vi "PDF HovaCAL fix Tables.vi"(8 "Sprachliste":string[][](array[string])) -> (2 "Bemerkungen":string[](array[string]), 3 "Eingabetabelle behandelt":string[][][](array[string]))   [LabVIEW 2020, in "Linearisierung v2.lvlib" / "Protokoll.lvlib"]
uses:
  Protokoll.lvlib
  Gasteiler/HovaCAL_Interface/Kommunikation/Aktion FGV HovaCAL Interface Autolin.ctl
  Visualisierungs Elemente/String - Ausgabefeld.ctl
  Seiten/FT-IR/FGV FT-IR Gasliste Aktionen.ctl
  Aktion Lin Daten aufarbeiten.ctl
  Gasteiler/HovaCAL_Interface/Kommunikation/Kommunikation.lvlib
  Seiten/FT-IR/FT-IR.lvlib
  Gasteiler/Gasteiler.lvlib
  Gasteiler/HovaCAL_Interface/Helper/Helper.lvlib
  Sprachverwaltung/Sprachverwaltung.lvlib
  Linearisierung v2.lvlib
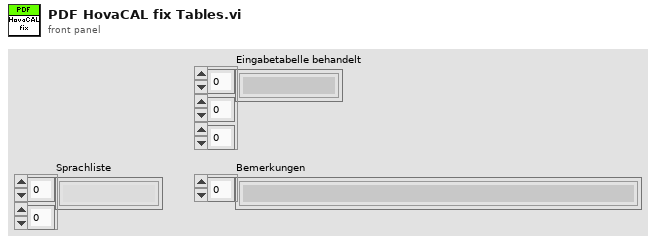
[diagram p1: front panel]
types:
  T1 = typedef "String - Ausgabefeld.ctl" = string
  T2 = typedef "Linearisierung v2.lvlib/Gasteiler.lvlib/HovaCAL_Interface.lvlib/Kommunikation.lvlib/Aktion FGV HovaCAL Interface Autolin.ctl" = enum16{"lesen", "schreiben", "MFC Komponente fix setzen", "init"}
  T3 = typedef "Linearisierung v2.lvlib/Aktion Lin Daten aufarbeiten.ctl" = enum16{"lesen", "Protkolldaten", "speichern", "laden", "EPA auswerten", "Tabelle schreiben", "Lin auswerten", "Tab init", "Stufentabelle", "EPA aktiviert", "Nachbehandlung laden", "Tabelle löschen", "Istwerte löschen", "Zeile löschen", "Zeile einfügen", "LIN aktiviert", "LIN/EPA aktiv laden", "EGAK Tab", "LIN übernehmen", "Tab init ohne Stufen"}
  T4 = typedef "FT-IR.lvlib/FGV FT-IR Gasliste Aktionen.ctl" = enum16{"lesen", "Gasliste FT-IR", "Gasliste ausgelesen", "laden", "speichern", "löschen"}
  T5 = typedef "Linearisierung v2.lvlib/Eingabetabelle.ctl" = string[][]
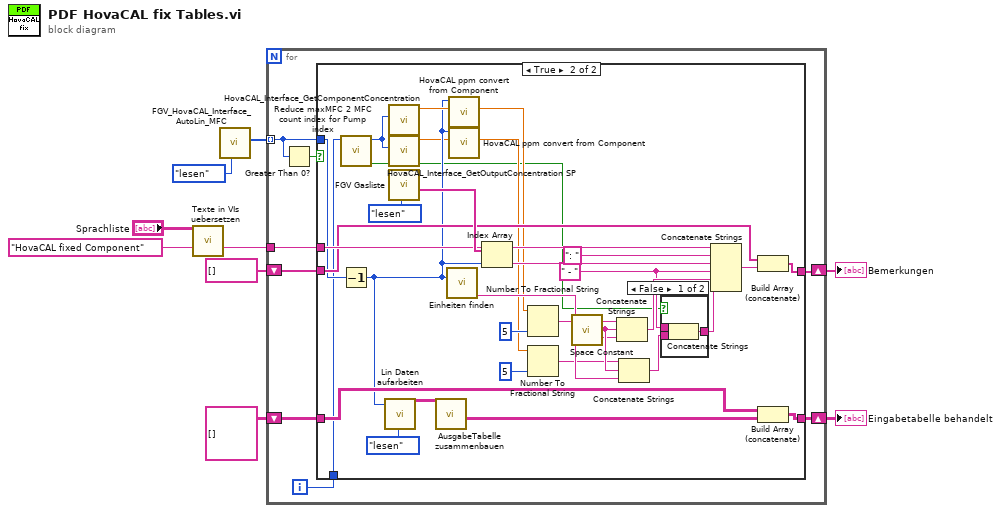
[diagram p0: block diagram]
diagram:
  n1 = call "Texte in VIs uebersetzen.vi"("Sprachliste"="Sprachliste", "String zum Übersetzen"=T1 "HovaCAL fixed Component" ("String")) -> ("String zum Übersetzen"=w6:string)  [unwired: 9 in, 4 out]
  n2 = call "FGV_HovaCAL_Interface_AutoLin_MFC.vi"("Aktion"=Aktion_FGV_HovaCAL_Interface_Autolin."lesen") -> ("MFV Komponente fix out"=w8:u16[])  [unwired: 7 in, 3 out]
  n3 = for {
    tunnel: w8 -> [w16] mode=indexing
    tunnel: w6 -> [w15]
    shift-right: [w14] -> w4
    shift-left: string[] [] -> [w13]
    shift-right: [w12] -> w1
    shift-left: string[][][] [] ("Eingabetabelle behandelt") -> [w11]
    i -> [w10]
    n4 = Greater Than 0?(x=w16) -> (x > 0?=w17:bool)
    n5 = case shown="True" w17 {
      tunnel: w16 -> [_ w30]
      tunnel: w15 -> [_ w40]
      tunnel: [w19 w38] -> w14
      tunnel: w13 -> [w19 w37]
      tunnel: [w18 w32] -> w12
      tunnel: w11 -> [w18 w31]
      tunnel: w10 -> [_ w29]
      frame False {
      }
      frame True {
        w22 = " - " ("String")
        n6 = call "Reduce maxMFC 2 MFC count index for Pump index.vi"("MFC idx"=w29) -> ("Pump"=w21:bool, "AutoLin MFC"=w49:i32)  [unwired: 8 in, 1 out]
        n7 = Decrement(x=w30) -> (x-1=w27:u16)
        n8 = call "Lin Daten aufarbeiten.vi"("Index (Seite)"=w27, "Aktionen"=Aktion_Lin_Daten_aufarbeiten."lesen") -> ("Eingabetabelle"=w34:T5)  [unwired: 15 in, 10 out]
        n9 = call "HovaCAL_Interface_GetComponentConcentration.vi"("AutoLin MFV Index"=w49) -> ("Konzentration"=w28:dbl)  [unwired: 8 in, 2 out]
        n10 = call "HovaCAL_Interface_GetOutputConcentration SP.vi"("AutoLin MFC Index"=w49) -> ("Konzentration"=w25:dbl)  [unwired: 8 in, 2 out]
        n11 = call "FGV Gasliste.vi"("Aktionen"=FGV_FT-IR_Gasliste_Aktionen."lesen") -> ("Aktuelle Gasliste gesamt"=w51:T1[])  [unwired: 8 in, 2 out]
        n12 = call "AusgabeTabelle zusammenbauen.vi"("Eingabetabelle"=w34) -> ("Eingabetabelle behandelt"=w33:string[][])  [unwired: 8 in, 2 out]
        n13 = call "Einheiten finden.vi"("Komponente"=w27) -> ("Einheit in String"=w47:string)  [unwired: 6 in, 4 out]
        n14 = call "HovaCAL ppm convert from Component.vi"("Konzentration"=w28, "Gasnummer"=w27) -> ("Konzentration in %"=w26:dbl)  [unwired: 5 in, 4 out]
        n15 = call "HovaCAL ppm convert from Component.vi"("Konzentration"=w25, "Gasnummer"=w27) -> ("Konzentration in %"=w24:dbl)  [unwired: 5 in, 4 out]
        n16 = Index Array(array=w51, index=w27) -> (element=w43:T1)
        n17 = Number To Fractional String(number=w26, precision (6)=i16 5 ("Genauigkeit (6)")) -> (F-format string=w50:string)  [unwired: 2 in]
        n18 = Number To Fractional String(number=w24, precision (6)=i16 5 ("Genauigkeit (6)")) -> (F-format string=w44:string)  [unwired: 2 in]
        n19 = call <vilib>:"Space Constant.vi"() -> ("String"=w48:string)
        n20 = Concatenate Strings(w50, w48, w47) -> (w41:string)
        n21 = Concatenate Strings(w44, w48, w47) -> (w23:string)
        n22 = case shown="False" w21 {
          tunnel: w23 -> [w54 _]
          tunnel: w22 -> [w53 _]
          tunnel: [w52 _] -> w20
          frame False {
            n23 = Concatenate Strings(w53, w54) -> (w52:string)
          }
          frame True {
          }
        }
        n24 = Concatenate Strings(w40, T1 ": " ("String"), w43, w22, w41, w20) -> (w39:string)
        n25 = Build Array (concatenate)(w37, w39) -> (w38:string[])
        n26 = Build Array (concatenate)(w31, w33) -> (w32:string[][][])
      }
    }
  }
  "Bemerkungen" <- w4
  "Eingabetabelle behandelt" <- w1
